vi "Grid_Create.vi"(0 "reference":refnum<class "Grid.lvclass">, 1 "gridColor":u32(colorbox), 5 "error in (no error)":errorcluster, 6 "GoopReferenceIn":T1) -> (14 "reference out":refnum<class "Grid.lvclass">, 16 "# of objects":i32, 19 "error out":errorcluster)   [LabVIEW 2014, in "Grid.lvclass"]
doc: "Creates and initializes a new Grid object.\n\nThis object should be destroyed using a Grid destructor VI.\n\n[GOOP 2.1]"
uses:
  <resource>/Framework/Providers/Open_GDS/UML/Grid_class/Grid.lvclass
  <resource>/Framework/Providers/Open_GDS/UML/Grid_class/ObjectReference.ctl
panel:
  # "The input reference should only\nbe wired when this method is called\nby a sub class constructor."
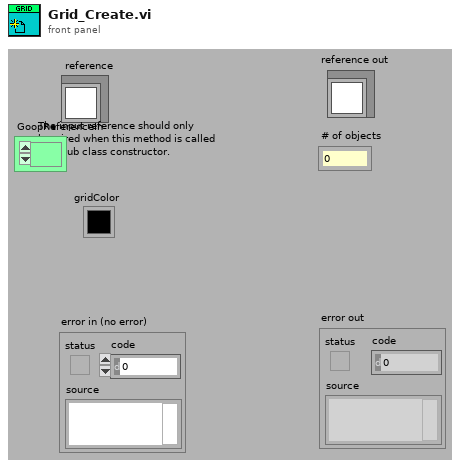
[diagram p1: front panel]
types:
  T1 = typedef "Grid.lvclass/ObjectReference.ctl" = refnum<k1>
  T2 = typedef "Grid.lvclass/ObjectAttributes.ctl" = cluster{"gridX":dbl, "gridY":dbl, "gridColor":u32}
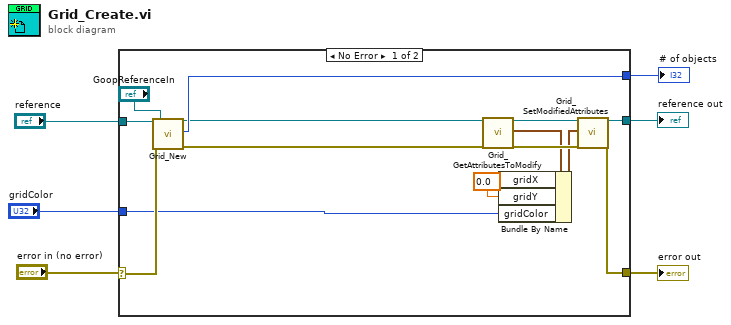
[diagram p0: block diagram]
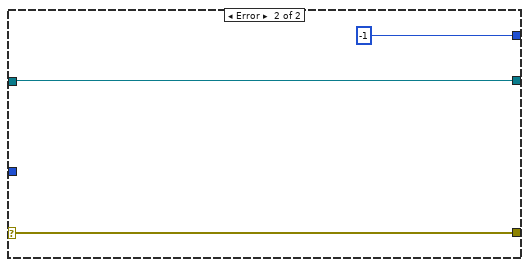
[diagram p2: hidden frame]
diagram:
  n1 = case shown="No Error" "error in (no error)" {
    selector: "error in (no error)" -> [w20 w22]
    tunnel: [w15 w21] -> w6
    tunnel: [w18 w22] -> w5
    tunnel: [w19 -1 ("Nr of open handles")] -> w4
    tunnel: "reference" -> [w14 w21]
    tunnel: "gridColor" -> [w8 _]
    frame No Error {
      w9 = 0.0 ("gridX")
      n2 = call <resource>:"Grid_New.vi"("reference in"=w14, "error in (no error)"=w20, "GoopReferenceIn"="GoopReferenceIn") -> ("reference out"=w11:refnum<class "Grid.lvclass">, "# of objects"=w19:i32, "error out"=w10:errorcluster)  [unwired: 2 in, 12 out]
      n3 = call <resource>:"Grid_GetAttributesToModify.vi"("reference in"=w11, "error in (no error)"=w10) -> ("reference out"=w16:refnum<class "Grid.lvclass">, "Attributes"=w13:T2, "error out"=w17:errorcluster)  [unwired: 1 in, 14 out]
      n4 = Bundle By Name(cluster=w13, "gridX"=w9, "gridY"=w9, "gridColor"=w8) -> (w12:T2)
      n5 = call <resource>:"Grid_SetModifiedAttributes.vi"("reference in"=w16, "Attributes"=w12, "error in (no error)"=w17) -> ("reference out"=w15:refnum<class "Grid.lvclass">, "error out"=w18:errorcluster)  [unwired: 3 in, 12 out]
    }
    frame Error {
    }
  }
  "error out" <- w5
  "reference out" <- w6
  "# of objects" <- w4
